vi "Calibrate Probe Tube.vi"(9 "Left":string="ABI-R", 10 "Right":string="SN31", 11 "User ID":string) -> ()   [LabVIEW 2020]
uses:
  epl-vi-lib/Utility VIs/Type Defs/Left-Right ring.ctl
  <vilib>/printing/EasyPrintingControls.llb/layout_options.ctl
  <vilib>/printing/EasyPrintingControls.llb/orientation.ctl
  <vilib>/printing/EasyPrintingControls.llb/panel_scaling_for_page.ctl
  <vilib>/printing/EasyPrintingControls.llb/margins.ctl
  <vilib>/printing/EasyPrintingControls.llb/margin_values.ctl
  <vilib>/printing/EasyPrintingControls.llb/measurement_system.ctl
  <vilib>/printing/EasyPrintingControls.llb/printer_options.ctl
  <vilib>/printing/EasyPrintingControls.llb/printing_method.ctl
  <vilib>/printing/EasyPrintingControls.llb/color_or_monochrome.ctl
  <vilib>/printing/EasyPrintingControls.llb/page_header_options.ctl
  <vilib>/printing/EasyPrintingControls.llb/page_headers.ctl
  <vilib>/printing/EasyPrintingControls.llb/page_header_content_options.ctl
  Type Defs/ACal-Probe Tube Parameters.ctl
  Type Defs/Cal Stimulus.ctl
  <vilib>/printing/EasyPrintingControls.llb/contents.ctl
  epl-vi-lib/Utility VIs/Math VIs/FFT x(t) to dB,Degrees (2D).vi
  epl-vi-lib/Utility VIs/Conversion VIs/Create Waveform Cluster (2D).vi
  SubVIs/Calibration Globals.vi
  <vilib>/printing/EasyPrinting.llb/Easy Print VI Panel or Documentation (refnum).vi
  Instance           1 28Saved   Calibrate Probe Tube .vi
  epl-vi-lib/Utility VIs/Math VIs/dB to Linear (scalar).vi
  <vilib>/Utility/NIReport.llb/NI_ReportGenerationCore.lvlib
panel:
  in  "layout options":T1={"orientation (unchanged)"=0, "panel scaling for page (unchanged)"=0, "margins"={"override VI margins (false)"=FALSE, "margins (1.00)"={"top"=1.0, "left"=1.0, "right"=1.0, "bottom"=1.0}, "measurement system (default)"=0}, "printer options"={"destination printer name (current)"="", "printing method (unchanged)"=0, "color or monochrome (unchanged)"=0}, "page header options"={"page headers (unchanged)"=0, "page header content options"={"Include VI Name"=TRUE, "Include VI Path"=TRUE, "Include Last Modification Date"=TRUE, "Include Date Printed"=TRUE, "Include Page Number"=TRUE, "Include VI Icon"=TRUE}}} {"page header options"."page headers (unchanged)" items=["Unchanged", "Include page headers", "Do not include page headers"]; "printer options"."color or monochrome (unchanged)" items=["Unchanged", "Color/grayscale", "Monochrome"]; "printer options"."printing method (unchanged)" items=["Unchanged", "Standard", "PostScript", "Bitmap"]; "panel scaling for page (unchanged)" items=["Unchanged", "No Scaling", "Scale front panel to fit"]; "orientation (unchanged)" items=["Unchanged", "portrait", "landscape"]; "margins"."measurement system (default)" items=["Default", "US", "Metric"]; "margins"."margins (1.00)"."right" format="%.2f"; "margins"."margins (1.00)"."bottom" format="%.2f"; "margins"."margins (1.00)"."top" format="%.2f"; "margins"."margins (1.00)"."left" format="%.2f"}
  in  "Correction curve":path
  in  "Measure":bool
  out "(mV/Pa)":dbl=40.0 format="%#_4g"
  out "Acoustic System ID":string="SN31"
  in  "Ear":T13
  in  "Probe Mic Gain (dB)":dbl
  in  "Cal Mic Gain (dB)":dbl=40.0
  in  "Stimulus":T14={"Min Freq (Hz)"=50.0, "Max Freq (Hz)"=50000.0, "Freq Step (Hz)"=50.0, "Waveform"=enum."Chirp", "Attenuation (dB)"=30.0, "Sample Rate (Hz)"=100000.0}
  out "Stimulus graph":cluster{i32, dbl, dbl[]}(graph)={0, 0.01, [-5.247460171907412, 0.008605798542191699, -5.263937532639148, 0.024339294749305594, -5.244475767281008, 0.04327175038935926, -5.188768276233243, 0.07159908666817012, -5.095903568565098, 0.11549515149058191, -4.964399941130261, 0.1810884237842581, -4.792264316991073, 0.27442378081433927, -4.577077172797298, 0.40140354945941514, -4.3161060418071555, 0.5677023140763962, -4.0064504089795046, 0.7786503888896317, -3.645220836759635, 1.0390815630417642, -3.2297547859327076, 1.3531417859996795, -2.7578707294700084, 1.724056982991224, -2.22816070014333, 2.153860279401379, -1.6403192706341323, 2.643081666319236, -0.9955040585896162, 3.1904066322148728, -0.2967191285234929, 3.792314555323266, 0.4507918747408072, 4.442712676082995, 1.2391613126860297, 5.132587144315406, 2.057546184165045, 5.849698747965765, 2.8918403003749833, 6.5783571298986745, 3.724486549481605, 7.299313078445633, 4.534431115953833, 7.989813153488007, 5.297265336532347, 8.623863622799167, 5.985602242560379, 9.172750412799761, 6.5697326691648446, 9.605857387646246, 7.018598937096457, 9.891815588212754, 7.301111383534703, 10.0, 7.387813446513752, 9.902367138660988, 7.252873956718745, 9.575595866011744, 6.876350702602797, 9.003455705946067, 6.246627988988914, 8.179282815334176, 5.362884683208197, 7.108396197100778, 4.237401343653944, 5.810239657287673, 2.8974701412652104, 4.3199938484742715, 1.3866355939228834, 2.6893743744841005, -0.235024890715656, 0.9863243167635698, -1.8918657346432832, -0.7066688960181444, -3.49512904116343, -2.2958437123541913, -4.947057814678465, -3.6811314381434963, -6.146708184335848, -4.762782149907513, -6.99733253447503, -5.44942121944958, -7.414996574301741, -5.667084312081226, -7.3378591109482, -5.368539628350952, -6.735306113447965, -4.541978733119788, -5.615921799386064, -3.2179767099964502, -4.033137435294095, -1.4735296001117006, -2.0873657499853566, 0.5679853545614835, 0.0764536954682828, 2.7418756260149975, 2.2766729673521082, 4.8527764144117835, 4.30839594053929, 6.690828848153954, 5.96217634437059, 8.052592456156836, 7.04673009875188, 8.765032133153767, 7.413566916427472, 8.710067062700757, 6.980647540350419, 7.846463408719186, 5.751601312013723, 6.225456709762098, 3.826859567750187, 3.9965653470462574, 1.4034232691160335, 1.4007322096543322, -1.2390126171416238, -1.2507325298668845, -3.7661990085581607, -3.6109846093868825, -5.830158904497616, -5.343446619696167, -7.11863088939354, -6.173269096842483, -7.406665287984586, -5.93697567074002, -6.602097328524571, -4.62149439465155, -4.7759155920390555, -2.383800918156967, -2.1693905978568395, 0.4558663898494483, 0.8275208795869367, 3.4507072628822213, 3.7275911979607788, 6.09235566166205, 6.022996250896586, 7.896571926877759, 7.276660398539333, 8.496267869824582, 7.212524412699896, 7.724300184680044, 5.78609054729564, 5.667189460480745, 3.217206541451461, 2.6736060915361497, -0.028096090734308465, -0.6915362170521967, -3.3109044902910116, -3.7458551362852015, -5.9401233137836575, -5.8269949248777975, -7.320204962233645, -6.442849713395074, -7.095298209127541, -5.400691974640072, -5.2545546954009525, -2.8805696820323017, -2.1668301265948715, 0.5736091158430698, 1.4744009601043935, 4.155120373461428, 4.794822743297185, 6.9746253410301975, 6.946647025249635, 8.282863836240622, 7.332782067475395, 7.681230357484651, 5.788485263093952, 5.259985350440268, 2.6635543896510905, 1.6148842229039682, -1.2321309711394293, -2.2791036731398298, -4.822173581640922, -5.318706845785659, -7.056875219949377, -6.58844576757031, -7.229540772397591, -5.652758866191721, -5.220125424480435, -2.728934669369589, -1.5792762725530691, 1.330004185915103, 2.5947767617377417, 5.26077489392688, 5.97156978417373, 7.7740442713520075, 7.413058271139368, 7.985588198248131, 6.374378980649487, 5.749844302517612, 3.1368042021591003, 1.7656193472640005, -1.2307138864244704, -2.6113675396896427, -5.199351313853099, -5.814263689192346, -7.309114034900627, -6.631386968823555, -6.720768410023753, -4.6897473313856715, -3.5800621548930938, -0.6575552182543789, 0.9704821464587078, 3.946321771794807, 5.176186930576256, 7.302284923331499, 7.337662376963383, 8.011803580119759, 6.514041666961232, 5.706545139116614, 2.967861932299919, 1.272343162390996, -1.8678232780009332, -3.45026885495027, -5.936024879819881, -6.411238921879773, -7.425541450334893, -6.252421914203625, -5.60197735072843, -2.9681759541147814, -1.212009047625889, 2.0072496296359597, 3.7722442843035657, 6.384557487487479, 7.0125100927973065, 8.061414715811145, 6.909383622455292, 6.155974853894271, 3.4311420962567754, 1.5162174765733274, -1.7766786708006803, -3.603327988185656, -6.125870985627785, -6.610596375301682, -7.3634425246130135, -5.9022705997704525, -4.770419048180873, -1.766887564352594, 0.3676255453902768, 3.661744223349101, 5.341314962064073, 7.462373475230487, 7.424660487516245, 7.498419729909054, 5.39409958927202, 3.6620769715753356, 0.30429290403609865, -1.9527130941819373, -4.9937392207499105, -6.143652224116909, -7.419717721833314, -6.423937846193488, -5.477259487880406, -2.545241904374176, -0.2381215906009224, 3.2334674915729873, 5.176970492062233, 7.403858060906316, 7.424812063901678, 7.332703585945119, 5.029648312147353, 2.9739938247968354, -0.5802426219546769, -2.96980091563933, -5.8492898574021845, -6.669677540664699, -7.320605771962078, -5.64372583856975, -3.941020091557808, -0.486803126553241, 2.1098537508064745, 5.382645863920707, 6.752794304321151, 7.939975165779068, 6.746137374430747, 5.3354630175248, 2.0049498872310276, -0.6926053124611669, -4.188393767139286, -5.895140320125075, -7.396021670989176, -6.4835405802843695, -5.2183372128746655, -1.9420199456520648, 0.8323095237238995, 4.436623036483066, 6.288347883410518, 7.866933818470105, 6.992701149290664, 5.66877018952909, 2.3174894102616133, -0.5588466061601974, -4.1880383393350575, -6.003821804112207, -7.419019451098028, -6.328409829492962, -4.734284432309863, -1.1850596867744247, 1.7950178654578355, 5.327091429463836, 6.882140261576732, 7.856640472116676, 6.2803281835987645, 4.22068034616256, 0.3991421081048472, -2.6140204156880023, -5.848350195807402, -6.85636573457159, -7.0910659692341325, -4.7933509719516, -2.1643551542287414, 1.8675265370492249, 4.689874030204529, 7.292308668251718, 7.390111510847516, 6.59199906715598, 3.4336871141493432, 0.30172855553474925, -3.673492374680839, -5.894931811807184, -7.418729223490227, -6.245322255897431, -4.25209871294359, -0.3328874715123917, 2.941917812152746, 6.31946557919589, 7.353133838306091, 7.330124735659604, 4.678678601940708, 1.6295522117378556, -2.5755880072377595, -5.28712450014373, -7.3144555947664305, -6.5735977356081134, -4.770194836178391, -0.8591488588596867, 2.5958602653035596, 6.156976691276675, 7.339590352317998, 7.295293625358333, 4.53266183919819, 1.2891964301376782, -3.0072298175380503, -5.6738166720809495, -7.406990997361928, -6.239496306224862, -3.941192684323301, 0.28294268668459244, 3.772424756570202, 6.9388943995771974, 7.412642145914989, 6.459663864604533, 2.929223388058357, -0.7253749311016806, -4.816256232005783, -6.702620432750113, -7.192902344033079, -4.731369021984241, -1.4414577990167237, 3.0487448569867754, 5.973294402720529, 7.777452265528625, 6.517475422558797, 3.929398783800692, -0.5311427078538121, -4.102206564584618, -6.975532546438933, -6.877235917573633, -5.151749627809858, -1.019946035576886, 2.85574857117119, 6.5142866732599245, 7.426122482652017, 6.575512793162643, 2.9296826424821316, -1.0056189595996894, -5.194472124415492, -6.9244564830663755, -6.869539692795811, -3.7564721469176305, 0.08751061193103099, 4.601488283996679, 6.950180666067047, 7.552463858896631, 4.928522407334323, 1.2339857195152837, -3.467697768024356, -6.260941260422518, -7.362010266767195, -5.130404817874262, -1.5787085489641972, 3.2260063318414076, 6.312999422865575, 7.742481983040587, 5.765824502092311, 2.29686139113806, -2.574183972128345, -5.832423189894068, -7.423361194717821, -5.547501807955327, -2.0757399684555327, 2.8460977007969532, 6.161201434600137, 7.740164989978125, 5.795240360236828, 2.218825065094677, -2.7480716752965813, -6.007130819195174, -7.397987435336653, -5.214791695268458, -1.4420055667696872, 3.5441107546488215, 6.610757652541965, 7.62161758419931, 5.032758273140988, 0.9938080906391938, -3.951552010030123, -6.6595244673234735, -7.090866741949985, -3.9541424698949124, 0.3666032462722816, 5.147025662921905, 7.283044503087227, 6.928843038131749, 3.143361282651853, -1.4005374850137773, -5.81753201637329, -7.131470601307786, -5.810562685267453, -1.3593972322635997, 3.237678001181557, 7.002954174075119, 7.220586802896102, 4.810421693830754, -0.2037693220285648, -4.557771783842997, -7.313595030973062, -6.190231619270408, -2.694006520878864, 2.6098313187672977, 6.2881002013277385, 7.644888179741437, 5.0332073532217505, 0.6422276509988876, -4.487733612052248, -6.96433742668024, -6.595428622107091, -2.5521855587978552, 2.2865678633506223, 6.597316176229779, 7.338285239994512, 5.1022254419284385, -0.016959372200316996, -4.591293583267117, -7.350470455953657, -5.978220674993969, -2.0764227867177043, 3.395236816869554, 6.791143158965057, 7.352228162218951, 3.8427701774074103, -1.0672643055181525, -5.8459021684587515, -7.149031971945431, -5.219227891725583, -0.1004177592343227, 4.6887830076421055, 7.5990316517010985, 6.2070269269780445, 2.115688988887157, -3.4661362625146603, -6.731658881182953, -6.8519111390977505, -2.8522801918666163, 2.2862242384436673, 6.72900730089474, 7.220900563595496, 4.35586130070044, -1.2229073577912795, -5.648862915611157, -7.389024632985817, -4.615740146897012, 0.31918760965121495, 5.5837098321905545, 7.426544277044912, 5.664192513987078, 0.4030823548800622, -4.600945112795148, -7.394431544905614, -5.557595320391062, -0.9370090027809214, 4.704655561012707, 7.339889092334802, 6.2787112720154, 1.2827129427791721, -3.979843266775962, -7.296417113586281, -5.922507567322214, -1.44318806531093, 4.356269929683986, 7.283021687223988, 6.4054972254029865, 1.4203851555677962, -3.947198285633883, -7.304928863219976, -5.849233412081237, -1.2139889713487029, 4.617712545093255, 7.353534406789328, 6.100063253697727, 0.8216317054554423, -4.511552759408483, -7.406095318826852, -5.304382372452656, -0.2405691394206577, 5.428240566118344, 7.425926703045357, 5.243465598093195, -0.5279946590706618, -5.533588570328488, -7.361872248281549, -4.096618104825187, 1.474264963016517, 6.551434833095712, 7.150728253852704, 3.5971745791139096, -2.5716981435457846, -6.655679885547709, -6.719722629272131, -1.9809781668597604, 3.7704867106062423, 7.484853597327619, 5.995321810252248, 0.9693345027842137, -4.9883959449077615, -7.21701623238748, -4.913340447389673, 1.1014843094368336, 6.1077362733100005, 7.418653590903101, 3.4379736602408677, -2.469318380430274, -6.9739072004505465, -6.306633286082643, -1.5808149986014717, 4.647425939667652, 7.407876735275789, 5.4427259675944075, -0.5738915711179777, -5.795510780887788, -7.226577076684699, -3.1818117873187712, 2.853476296586651, 7.275652090831912, 6.283712090560184, 1.2100048808955002, -4.988063124485182, -7.225270522900655, -4.5176796337619365, 1.8444352873823244, 6.631109219631903, 6.992678228704494, 2.0109920015762643, -4.063299376258122, -7.405929161515044, -4.916771011045486, 0.9678524128825984, 6.522515137830295, 6.99560041193589, 2.6271152187851907, -3.948885437252043, -7.192300800581729, -5.2534136062223, 1.0318439544846199, 6.311848705567506, 7.166209195204141, 2.323350785231853, -3.936826451465734, -7.405888659140412, -4.805723062168871, 1.290124743453395, 6.75573752449112, 6.749821833712563, 1.835291400009754, -4.741122013944317, -7.242224259477733, -4.254776132185593, 2.456246771732051, 7.013090118914596, 6.349145545303646, 0.4051417927954177, -5.5188544634287195, -7.226690557563207, -2.765024839084136, 3.729343570414043, 7.554573672535005, 5.035548016008795, -1.2497620581093263, -6.722345116231772, -6.341040872374437, -0.938777516835575, 5.584937372087172, 7.29088401898383, 3.277752823374007, -3.668197539629081, -7.21954700648047, -4.9141953866504275, 1.8607845337324562, 6.881419700776224, 6.414705610677603, 0.3124143648746709, -5.733833290366328, -7.077455525208768, -2.0334400691400996, 4.577687291061455, 7.575544132680769, 3.845466604947863, -2.900155243337663, -7.312647657904366, -5.0325387969350555, 1.4726554460206769, 7.010693797557449, 6.208835270027705, 0.2426368501627138, -6.119786289628639, -6.742878807224529, -1.5366022807910058, 5.358562178640916, 7.291008275054191, 2.986361087280685, -4.181914869472955, -7.27254284643081, -3.9445461493243212, 3.276059924149099, 7.353406806436564, 5.017532453194594, -2.0827734646331777, -6.974967011951131, -5.603801799805588, 1.2479935717871624, 6.790144240279283, 6.3212911871910835, -0.19962218586423452, -6.245716249946395, -6.596693444669236, -0.4520652452418208, 5.971090033733906, 7.044081935464482, 1.2857370221473308, -5.4125325086995915, -7.105320196586026, -1.7178422467752026, 5.1740674229367825, 7.380757371982751, 2.324840249908939, -4.701914033774923, -7.319981402284617, -2.5414947549511457, 4.577072426551161, 7.504757775455616, 2.935040678634225, -4.248566017694976, -7.389068349975114, -2.9525810734921025, 4.277627161008861, 7.534354087203025, 3.1477895890718384, -4.118723423292581, -7.3978556128306145, -2.97682477387077, 4.315562896229031, 7.520352295898593, 2.978030728532146, -4.329172031133085, -7.362041055431735, -2.6157810360379234, 4.686140136961194, 7.443176669474266, 2.413668319234095, -4.853212361187332, -7.226983660393568, -1.8457858961590197, 5.33833667896169, 7.213830229532318, 1.4239626016719844, -5.611417991409709, -6.870925073661793, -0.6360621551866662, 6.158908268204798, 6.680868903172948, -0.012198893040158035, -6.4506233835836015, -6.118102470078314, 1.012431405730744, 6.948896592720228, 5.652805457530667, -1.8568674591179255, -7.121721760234774, -4.774119857796032, 3.007873164854061, 7.407847897177656, 3.950236955566206, -3.9466082818682264, -7.2768739195418695, -2.698095427984128, 5.09842422101464, 7.151880583544878, 1.4998433771111057, -5.9280034587624915, -6.517113218616011, 0.08227476144176188, 6.823062584347205, 5.799336511097809, -1.5342933632456348, -7.237851950393849, -4.522792310107686, 3.233444877508748, 7.537944689067077, 3.148759997984469, -4.624501162666625, -7.193663995647283, -1.274986138271457, 6.025253604588409, 6.58732564498896, -0.5703477954587108, -6.855121697511509, -5.255351399441133, 2.6912635594559378, 7.407826844331432, 3.6548593814698234, -4.483060427885582, -7.134453506819222, -1.447213075625703, 6.166117630160645, 6.383081700870901, -0.7861948037197607, -7.105684033559456, -4.730501596501017, 3.233059875754157, 7.522314740973714, 2.67761848243742, -5.200149255925657, -6.871311330089527, -0.011331621791488056, 6.789393984493315, 5.520727292913766, -2.5675094974361627, -7.3215384228731555, -3.169811702407082, 5.078118913958271, 6.996959773882328, 0.4635379712645482, -6.720929830813573, -5.3743273661307756, 2.5898280055884793, 7.51816284613278, 2.9796279606995535, -5.107951957867861, -6.853606575165182, 0.2145104988875672, 6.948469445520113, 5.082335764255203, -3.2948186891216396, -7.307763003702785, -2.081545339836511, 5.986008904559052, 6.335270153507825, -1.2601441461697336, -7.3037108572907, -3.76436647820519, 4.575386453236491, 7.174988426803019, 0.40886276693731716, -6.718500000770266, -5.156288906754431, 3.3127785405012187, 7.392157940194016, 1.9481390390104314, -6.117936957570988, -5.958154081040177, 2.0133387073918496, 7.4921389318317395, 2.980132608481309, -5.330452107764856, -6.597880522116794, 1.108780699565278, 7.282270450218552, 3.85410194661178, -4.8092811093465295, -6.837333409733931, 0.31368410046975775, 7.203334999165943, 4.277662492602619, -4.3056702174620405, -7.078412185454286, -0.03438186957498213, 7.011907531884418, 4.602962511361689, -4.179018451126646, -7.058557225575194, -0.2457963493496157, 7.06140341649829, 4.540389278552674, -4.138530549108562, -7.106121206873734, -0.015365853308301175, 7.056711255870985, 4.393121269506496, -4.481737357836458, -6.911329938301271, 0.3598426758007237, 7.2690650721030785, 3.8489605944825476, -4.89245298687628, -6.721818960510642, 1.1651210279975381, 7.353013513759481, 3.1608890494445325, -5.6036906401199715, -6.184089002672798, 2.1021341308880115, 7.493896595507685, 2.0161520342524835, -6.251984549771036, -5.482094199600977, 3.3959908559018883, 7.291899898442843, 0.666279618824786, -6.971716416547719, -4.256797330499773, 4.683783173675891, 6.8555516801230185, -1.1236956068984163, -7.3188776276161445, -2.7005285739750873, 6.054328152527586, 5.771774923298172, -2.9959145246337897, -7.320499134142371, -0.5650429875992593, 7.011616036027911, 4.169076331702438, -4.983625449917584, -6.499797553302054, 1.7867319981344782, 7.484495672535726, 1.7913635809048556, -6.515479887937506, -4.9176851263388315, 4.306487294935299, 6.916154946198537, -0.9703314683939835, -7.393387655014362, -2.3237097363788646, 6.309106563315713, 5.298911133350756, -3.943825466303358, -6.961860452300179, 0.8234554913541505, 7.433342869355618, 2.4173152983473027, -6.278708931241014, -5.157599335555851, 4.165978845245447, 6.916269397202499, -1.1368038483555083, -7.417012847519947, -1.8608890143246493, 6.628569163314005, 4.685710151704879, -4.736484110149196, -6.510958460408045, 2.1010756992173847, 7.445750477929317, 0.8291057533600581, -7.02965646602411, -3.587187966152209, 5.735480122805063, 5.772359254023778, -3.4505655445327994, -7.092896487453685, 0.8836811297244362, 7.407655648134268, 1.9307107136610782, -6.719688658193731, -4.279548739125746, 5.170725786787521, 6.204679037376475, -2.996785318715991, -7.172596714740932, 0.49776084697882034, 7.426006530234811, 2.017631158258109, -6.66837225434066, -4.259696555741614, 5.336739235586457, 5.999907565678239, -3.3122677874397706, -7.0790578557442165, 1.130643519486488, 7.426867073907273, 1.2635949671344218, -7.048058314044763, -3.3520919032035184, 6.02307345106183, 5.230819827745236, -4.4800167570289915, -6.480778767262717, 2.5867974703342993, 7.293490166170975, -0.5198521180144519, -7.376174578741273, -1.5422206759324273, 7.016952559870459, 3.4449323971009664, -6.0290299939485195, -5.056927437130529, 4.761619679998125, 6.287895772338952, -3.0893308477577093, -7.079202239575908, 1.374775801813738, 7.414276063661718, 0.4919697724840566, -7.303053345831668, -2.1752733434697866, 6.787874814292458, 3.8020882523454325, -5.925106372577843, -5.087138350895923, 4.789833706094948, 6.18864210441624, -3.4575815730321158, -6.877426298905895, 2.010170539937892, 7.341581121149976, -0.5192665657090618, -7.401020568797851, -0.9455062464022865, 7.262813200154886, 2.330665799263958, -6.782728429921616, -3.5884637749515425, 6.172717552564091, 4.688957650630858, -5.3105372887895905, -5.607877755200963, 4.400303350121803, 6.337379392473475, -3.3307144254223697, -6.872944270575925, 2.2890559166616824, 7.223548472300287, -1.1680785719139684, -7.398264864377694, 0.1334415939306725, 7.416410018479477, 0.9209854360723804, -7.294296784950279, -1.8524520650484861, 7.0556901416999125, 2.765944521584717, -6.7189323138813, -3.5405505538122166, 6.3078322538462475, 4.2783293247911764, -5.839211019870375, -4.8779340722449085, 5.334209601773843, 5.4359950925258325, -4.806197163386051, -5.868145403133641, 4.272409227610091, 6.263089009181842, -3.7421169184660386, -6.551096798996301, 3.228486290643495, 6.810854343669898, -2.7369035091718157, -6.985435068214615, 2.276956012631502, 7.141965492640768, -1.8508271751906238, -7.235045328152592, 1.46532362307337, 7.319233862104875, -1.120278634308993, -7.359869430159808, 0.8205755195832674, 7.398364006797049, -0.5645229317121275, -7.410371912701982, 0.3558454834427866, 7.423874712291961, -0.19201220967215066, -7.424655369356793, 0.07618030599874454, 7.427157166498761, -0.005469421733202465, -7.427230463015562, -0.01714716141569475, 7.42575399924954, -0.0053761002394784535, -7.428634215170117, 0.07599364351345202, 7.423183005309935, -0.19173233891843405, -7.425362887881296, 0.35547256648551373, 7.4089212073272375, -0.5640576747585542, -7.3998878507086365, 0.8200189260273955, 7.35847182632419, -1.1196328593441274, -7.320831555676253, 1.4645915959194222, 7.233745459785213, -1.8500137808532942, -7.143687660520191, 2.2760675624765674, 6.984288856136283, -2.735949217361889, -6.812761209684803, 3.227477546164284, 6.550167413273623, -3.7410689909103785, -6.265244901517009, 4.27134025432215, 5.867496052705217, -4.805129973770331, -5.438459285250389, 5.333170283282182, 4.877616717905038, -5.83823069799834, -4.281142526192145, 6.306945050488885, 3.540590198072637, -6.718176876739951, -2.7691111567212734, 7.05510677865644, 1.8528274290289084, -7.293928528267814, -0.9244533752976082, 7.4162987415759165, -0.132818336985834, -7.398451730141151, 1.1644369953415918, 7.224068954342528, -2.288355223399794, -6.873828011689916, 3.3271136589993873, 6.338644297302056, -4.399782504607134, -5.609529600364011, 5.307273332538398, 4.690983798162676, -6.172703613171116, -3.590833312033117, 6.780147752037883, 2.333323888376624, -7.263656143383226, -0.948376032135294, 7.399456530337989, -0.5162875524339932, -7.343573759427886, 2.0072051922935303, 6.877104314241444, -3.4547732535611546, -6.19191412499727, 4.787336461080588, 5.088064593730297, -5.923080493918324, -3.806497651280201, 6.786472135171221, 2.1771391413601497, -7.302408840932891, -0.4970322216789631, 7.4144898134942485, -1.3726265822772437, -7.080329883784682, 3.0844236539756817, 6.289931255332871, -4.760110006045242, -5.059797647129997, 6.025259581286349, 3.448486988188797, -7.017048997819728, -1.5462376697209068, 7.374405141929314, -0.515662877445445, -7.295859359789407, 2.5827723313479654, 6.481385192945382, -4.476517940242472, -5.235462646037644, 6.0204507306915565, 3.354643120470073, -7.046616127697511, -1.2696273237792064, 7.42681906050643, -1.127457940232792, -7.080495585247652, 3.306500997165923, 6.002766494492259, -5.334780914164535, -4.263747781980172, 6.664750626009611, 2.022480594483122, -7.426949012757776, 0.49263877679293694, 7.17235199964729, -2.9920030389433516, -6.209096050999331, 5.166905137167382, 4.282435540599078, -6.717382532006223, -1.9374669609565376, 7.407253702447325, -0.8796397991271134, -7.094554372923783, 3.444106102793002, 5.775939653753163, -5.733266194931018, -3.592253837019415, 7.026405408350863, 0.8349480400453515, -7.447737561133129, 2.09534544545967, 6.512304597813737, -4.731810644145896, -4.691959785589022, 6.62578766384903, 1.8654096452406224, -7.416694437351456, 1.129108339115356, 6.918579662084281, -4.162131840100958, -5.162231198965337, 6.2738377553254665, 2.4234912578716203, -7.434087491324242, 0.8168691413127844, 6.9625731321676385, -3.9381305832087077, -5.305175618692445, 6.305508388999558, 2.3287308778455165, -7.39273333221167, 0.9619683348921999, 6.918703016090921, -4.302183403773263, -4.922998417302366, 6.510675562341595, 1.7983364322760444, -7.485960450584175, 1.7796646687065727, 6.501756309519529, -4.978157283984076, -4.176730609481952, 7.009149341278814, 0.571052691676939, -7.321768717118409, 2.987504426221774, 5.776587877050262, -6.051253172668277, -2.7077435875394817, 7.316534680634138, -1.1159462505698252, -6.860213533626597, 4.677623140441568, 4.261808797028619, -6.968947336445471, -0.6758019546077514, 7.293437803342252, -3.390165972287008, -5.4876318472838115, 6.2461631977725816, 2.0241446125112845, -7.4954119353173665, 2.0940759522437595, 6.187167758336899, -5.598114292790371, -3.1701275033281733, 7.351797337504524, -1.1580580802763034, -6.725505313751188, 4.884481308744809, 3.8564603654920004, -7.268363258796754, 0.3509859330417606, 6.912882810353109, -4.474590682398902, -4.401919906179307, 7.053881749985286, 0.022988448800186856, -7.108773997326044, 4.129480344469301, 4.547697255690019, -7.059723053721764, -0.2551245805506439, 7.059680792385098, -4.171223699204117, -4.611945558386291, 7.008762407642546, 0.042470663314095713, -7.081315557630775, 4.2963933331143425, 4.285592968508252, -7.202048473201601, 0.3038923316421848, 6.839434863403917, -4.801739350059988, -3.864136012017699, 7.280300005462442, -1.100319512200232, -6.602501910121454, 5.322037732448754, 2.989447224049214, -7.492893646869789, 2.0034541893218076, 5.962668338777362, -6.112059145100089, -1.9596868346605159, 7.3931639559278555, -3.3047948125244133, -5.163874183028224, 6.712774702292517, 0.41948497251843697, -7.179651304541224, 4.566926328514163, 3.7721017633222043, -7.301742938608468, 1.247974714653711, 6.340961932698631, -5.9808100328068114, -2.0921150883882254, 7.307239632493462, -3.2848626127685425, -5.092066037197858, 6.944504984781181, -0.20474190955431903, -6.857948843428377, 5.098375833844543, 2.990053475182424, -7.519297579123885, 2.5790650682322824, 5.380641776032993, -6.715999006321392, -0.4766188663610665, 7.000863251799099, -5.070901008731789, -3.180442871449945, 7.3195245653301555, -2.5563852601331076, -5.530328479134261, 6.784541075758663, 0.021846766029578427, -6.875870748801165, 5.19020057592572, 2.6889310631973586, -7.524267826482181, 3.222047600888891, 4.738337868478731, -7.102092994604997, 0.7724403891886568, 6.389418263773441, -6.160387201523187, -1.459478075988101, 7.135769908395196, -4.4730101181799045, -3.6674390146075444, 7.4068998598456695, -2.680792754051274, -5.264378563255567, 6.8491697160324865, -0.5575064840759716, -6.595111165912422, 6.017658233787291, 1.2862991316369836, -7.196900286925187, 4.612915273325978, 3.1606725654779995, -7.539482019353017, 3.2215078866958375, 4.531700522411171, -7.234851524908173, 1.5197555563401193, 5.807722455458481, -6.818743669479842, 0.06874191811179253, 6.521738478319468, -5.919786523848885, -1.5147501872859683, 7.155568020219869, -5.089681973749451, -2.7109603599788237, 7.27667821145293, -3.934822470750932, -3.9636585033284337, 7.406825360953803, -2.9964038113230105, -4.78490694433085, 7.1170984144646665, -1.8431296498239582, -5.663768656202124, 6.943841635253259, -0.9996830447815409, -6.126239135094078, 6.44242538231895, 0.0022661839074547474, -6.689148614238921, 6.150758430711532, 0.6491137587774676, -6.876473690356764, 5.600597037938297, 1.438431378236845, -7.219716927533895, 5.32800788552948, 1.858656623567726, -7.230408849302793, 4.84061743918104, 2.4278729447225573, -7.447263467847703, 4.674399499851773, 2.6283900709131776, -7.3640282309582075, 4.315486817425743, 2.992045282935633, -7.523390082580188, 4.303019677466001, 2.989368019667606, -7.399202672469594, 4.104499863871741, 3.1618987508963645, -7.537176064176618, 4.264799022449545, 2.965399091516734, -7.39063683180584, 4.234314619589935, 2.949607691346328, -7.508249288816504, 4.564492323474465, 2.5549391062473332, -7.322675857688303, 4.688220682057052, 2.340168464155817, -7.385834829248802, 5.162403783463528, 1.732128463925866, -7.110055992690154, 5.400174794944171, 1.3019109227170205, -7.05163839036323, 5.9612505643602445, 0.46710003258039723, -6.6043089484332125, 6.235743883185024, -0.1829227657568783, -6.3320645085950025, 6.78331932492377, -1.2328061845999947, -5.614873557507866, 6.968691662259254, -2.0664648083747257, -5.031861790195274, 7.350986726369583, -3.2619903508673036, -3.9590863704478507, 7.27136238791224, -4.167636243486004, -3.0038333371520984, 7.294295183317757, -5.347603856785915, -1.553673636572424, 6.747862476502382, -6.109829647955342, -0.2617036301608677, 6.2184968509740735, -7.005329076788003, 1.4552699482895806, 5.043760944872093, -7.3095157960751225, 2.882386539798747, 3.86078493627221, -7.578060173790286, 4.5634885893059804, 2.0492093738664683, -7.08292207485835, 5.721307226434584, 0.3305956155972155, -6.426019657561329, 6.87451611844762, -1.84439975171717, -4.92796616455454, 7.216134662172068, -3.6521194269538917, -3.296042654826917, 7.294400492737467, -5.573654506029841, -0.9572913111545998, 6.348543917775765, -6.714350580421591, 1.2298238259910688, 5.04938878832608, -7.553945454293956, 3.7129464338939493, 2.7809817034388855, -7.231056372723618, 5.505106297311093, 0.42424361211661904, -6.361264831276551, 7.006737013250193, -2.439371902402299, -4.270596708720245, 7.241505567361612, -4.726164670376518, -1.8557306482234468, 6.757935482804603, -6.7480969586471, 1.2708184123790633, 4.81878599994673, -7.404389234655259, 3.918913357156455, 2.3421345932955466, -7.174422736038775, 6.3013486152791, -1.0135204245187428, -5.267512589575221, 7.188534157845813, -3.9318776684931467, -2.6475785675015215, 7.002344494894086, -6.513412931662251, 0.9477685116477176, 4.930013829280428, -7.404379701622458, 4.045094340786787, 2.0306593181891355, -7.002367279442268, 6.621835978662278, -1.8258397362624548, -4.534033458089634, 7.224602677252942, -4.97269404183121, -1.2320477316455334, 6.294781517920667, -7.270778122603829, 2.8341632946516633, 3.198978124750698, -7.231391423808875, 5.781593017575835, -0.5528605758650056, -5.459158003220313, 7.4063281953931135, -4.631871853515469, -1.601600262943367, 6.315389847394693, -6.966529773901621, 2.447850744710138, 3.4569861922628107, -7.425240673390551, 6.095444184751662, -1.0815069300039253, -4.929556591440002, 7.215639408353774, -4.972264895553426, -0.9924847782794413, 6.008185400083194, -7.4818575849958755, 3.7515742001815027, 2.000490718543498, -6.729073025424236, 6.64579440736328, -2.550936603096015, -3.6183706182232376, 7.156697145515479, -6.541256852987952, 1.4523963409777605, 4.1133142458405665, -7.364794926851754, 5.51789649365079, -0.505557176160088, -5.261523967685936, 7.426258928041062, -5.413546798120738, -0.263235157814853, 5.318053870586352, -7.4043596589994065, 4.492482678274301, 0.844352857034492, -6.115537395358456, 7.350280323270243, -4.6006069887787335, -1.2367253215057632, 5.8609954617576125, -7.3007165912202545, 3.92653119050302, 1.4431880652798892, -6.419893604268694, 7.2784158512998705, -4.338275415375522, -1.4661598110978695, 5.934118913683494, -7.291991563704478, 3.958950664748876, 1.305963864342815, -6.293925752666992, 7.336234811203122, -4.687123985852185, -0.9606126730331556, 5.570984052327365, -7.392161468057767, 4.581301695092964, 0.4270305896089277, -5.682073935741933, 7.4262938029902, -5.5683777501965395, 0.2950364452285744, 4.632540459249535, -7.391433011418179, 5.632586262553019, -1.1988740828766566, -4.377654612826481, 7.226579729538144, -6.718450445829406, 2.262858753334338, 2.8731247253419645, -6.861379048083197, 6.721788759174529, -3.4442429483303, -2.14114457261647, 6.220624200353356, -7.596652158882762, 4.669432578779883, 0.12387692375389034, -5.236992463434808, 7.149084332880998, -5.830382883881306, 1.0410380798767536, 3.8643120403514413, -7.361226465593431, 6.7808670309515096, -3.3737095944247493, -2.1007829704785723, 5.99045721807297, -7.34677816766543, 4.570498185601873, 0.008613672596484849, -5.1231358843378425, 7.342191617399275, -6.585259614011678, 2.2620478527090846, 2.574553805673502, -6.607273960670142, 6.9570939290320055, -4.467031622868547, -0.6696608618019022, 5.052324327106797, -7.649743843598196, 6.274158172352818, -2.5864289592375957, -2.7184277658270983, 6.201577041856491, -7.3089648517917825, 4.536286597181077, -0.17736446399596073, -4.8328595514011345, 7.226742983588233, -6.993014288537623, 3.2137210986872775, 1.3838896103754983, -5.827148554402899, 7.129947624107842, -5.800840769478473, 1.3729310187592958, 3.1676946513050668, -6.942410035578347, 7.277720324031, -5.127992439988434, 0.33957055186316665, 3.974855609274266, -7.098896736644328, 6.648556419109189, -3.928448266747144, -1.0224589472135093, 5.052834982863984, -7.627831099689657, 6.598212026349369, -3.5208177769270548, -1.469001455707609, 5.2316972628351, -7.400380144351477, 5.991093989831807, -2.7222982355420977, -2.247125274400901, 5.812594418939864, -7.7427233018528705, 6.145580670964048, -2.821265821434809, -2.102605496007431, 5.563161626582352, -7.424209577944001, 5.815177136752605, -2.5477237929533865, -2.3255424622827627, 5.783608358808926, -7.745679498267217, 6.298014094539757, -3.2012855156352287, -1.6065085533261036, 5.148197704668377, -7.3657296410551485, 6.246286236890397, -3.442330560665203, -1.2639417779734765, 4.949991585873638, -7.560775044882288, 6.939971191850884, -4.579261804509102, 0.05858411924960321, 3.779123600247425, -6.880518934336202, 6.917040353601821, -5.173614763480565, 0.9754609373700446, 2.956506600714473, -6.592912141972517, 7.4258189084584085, -6.499306327430656, 2.8285933864815798, 1.047396122123962, -5.1729490368667586, 6.882326856563093, -6.965310319077968, 4.077020492657918, -0.5015307010060882, -3.956922458816071, 6.531699352884887, -7.776811366439418, 5.955507236501781, -3.0222961221574667, -1.4708296934614629, 4.751648719123602, -7.200330384846797, 6.691981343928857, -4.7932614113136305, 0.6940370291419778, 2.956991366449558, -6.478487982384133, 7.41442217295258, -6.926029486606039, 3.746193231842714, -0.2539470394846976, -3.967021195040008, 6.251749853525533, -7.4046460924651285, 5.654604556031489, -2.979120396374964, -1.3211889697237222, 4.557025442790835, -7.308144738886594, 7.3348313379395815, -6.138848324146861, 2.5668157793901107, 0.8882457301232092, -4.79396810354764, 6.582694652151162, -7.308962004789193, 5.265573222339429, -2.54623072019011, -1.6619016600411323, 4.702996543496684, -7.34299820504679, 7.348679944072046, -6.301756301900259, 2.912937368325551, 0.362837300700869, -4.277992932439985, 6.257722311250287, -7.417090175268114, 5.876733812361009, -3.645787054978731, -0.33506782078237074, 3.461965963942266, -6.611286905350711, 7.393194842073476, -7.281372738476794, 4.664950328748116, -1.8374308885384962, -2.1951255396175178, 4.8146900090927485, -7.1006011117078724, 6.848978759475313, -5.828316029691708, 2.5829805203545937, 0.43158173613830925, -4.250149129708139, 6.297659381527943, -7.860910136874013, 6.869818954407151, -5.303798097092393, 1.7632278811122357, 1.2155574943688954, -4.759540178375289, 6.340122881958311, -7.417312754207814, 5.986144172937015, -4.16069442657965, 0.5246046416014631, 2.3489569747076167, -5.693929552737952, 7.003825084669513, -7.864691027681262, 6.270581742742224, -4.409792936038569, 0.7991170110753397, 1.97213524398193, -5.242113557016021, 6.49346196345197, -7.392805536911185, 5.876502286494598, -4.160505865130327, 0.6578267192883152, 2.0374763679515113, -5.362595272327349, 6.760241212561402, -7.941376744791632, 6.738615836392951, -5.358361147182795, 2.077192239968285, 0.5191192688925419, -3.9699143045716863, 5.661231585117198, -7.326320600203067, 6.659725626219334, -5.828032675361544, 2.9379742147542807, -0.5458802351538145, -3.0080158388942864, 5.055017893867966, -7.3481262513305845, 7.425119819950367, -7.391905633350139, 5.152052923029143, -3.20248238397998, -0.27288734698164785, 2.5754074887880556, -5.500754902496265, 6.434232200829689, -7.417890885677318, 6.127114162366173, -4.967673000031969, 1.9181756054066286, 0.33947319724950403, -3.695562055299864, 5.418308414317603, -7.512708357590764, 7.4243142218918905, -7.450335338192585, 5.31665400343499, -3.6308323615766187, 0.3321398230231999, 1.79914116656524, -4.7976635210734795, 5.917922990275773, -7.368061649105391, 6.600712569894668, -6.105486129243958, 3.5722882353210865, -1.74173015644146, -1.5533898200158465, 3.463083883106812, -6.181473966913003, 6.92255847897142, -8.063486649740032, 7.000574489191534, -6.362960118523379, 3.740975055094738, -1.9729599665011293, -1.2478633659399847, 2.998482256910706, -5.625837740919566, 6.264219153614564, -7.426596722780991, 6.398613544129925, -5.913844377509871, 3.4182159381994284, -1.8321580021758126, -1.3105004576865906, 3.0016636662514258, -5.735158441688524, 6.531739569970374, -8.019546640911276, 7.331994466370419, -7.286645112735421, 5.149556171457292, -3.9142671796692436, 0.9336116352886903, 0.6927158330188999, -3.612672995234601, 4.7137959754242935, -6.73658179371383, 6.6346571947790824, -7.302209593913814, 5.795068501449539, -5.172343584324118, 2.5762835163537656, -1.1934421917001579, -1.804468492654923, 3.171088355631257, -5.7793003656119355, 6.393784309414009, -7.996049229345152, 7.411060370892994, -7.762557498808378, 5.948958347728496, -5.231718365678255, 2.5590674075491497, -1.2933333636387538, -1.6165629767290817, 2.7611072801118337, -5.247271942913456, 5.670032540312404, -7.238248279520735, 6.585217567275997, -7.0446006808992525, 5.29561152171372, -4.792602259262475, 2.2425269594214385, -1.1938112847959148, -1.6549067841050247, 2.6998589046144614, -5.2927446310950454, 5.812870310423772, -7.698292293713049, 7.3388236732487755, -8.28019598300212, 6.932910914940819, -6.9534162389356515, 4.764972257948207, -4.121203823492364, 1.4360094015377518, -0.5357722872155042, -2.204341640419693, 2.9128690389473446, -5.282266228656416, 5.419591731393694, -7.106839860224447, 6.4438021304455715, -7.313059986369838, 5.809598972571791, -5.915965939957716, 3.713706626485786, -3.2749969843658926, 0.6512300911768543, 0.012026951770659284, -2.714019987392237, 3.253414807170112, -5.69991845017277, 5.8113132432249195, -7.743324131730205, 7.2220557533050425, -8.498380450091945, 7.268899630789249, -7.881800176248844, 5.99954486150076, -6.063748999136739, 3.692761927651043, -3.4136061127888384, 0.787414151244069, -0.41684012306177026, -2.2080310034069353, 2.41812472939367, -4.806846768252448, 4.645499889116734, -6.620531848055124, 5.946865109984115, -7.409905347313126, 6.167509800001608, -7.106322017952566, 5.322833865617136, -5.804172009452375, 3.578359262439368, -3.7302051938133314, 1.2104385444748584, -1.1978513115225842, -1.4435399239016196, 1.444467731214275, -4.03664782410229, 3.8627627119142764, -6.25815082231989, 5.778194335534294, -7.86819819366995, 6.995042836043658, -8.718691134212639, 7.414384035235543, -8.759938452079965, 7.034122922408689, -8.034654277369544, 5.937686580174754, -6.66218128204142, 4.27467462474421, -4.8164904448940336, 2.2371199399618695, -2.701575755643038, 0.03482568895657347, -0.5274594690958865, -2.1273331461358005, 1.5106872433618135, -4.068058156254445, 3.248659237728493, -5.643013827979403, 4.563778945895203, -6.752559806240499, 5.379874073549703, -7.344117745090801, 5.667232207973067, -7.4099562403169825, 5.438488776356751, -6.981474683255755, 4.741607705078281, -6.121181718514305, 3.651149172940014, -4.913528823321419, 2.258923894463806, -3.4556155395432104, 0.6649510738346807, -1.848572613500148, -1.0305914032602168, -0.1901912425558332, -2.733975688884164, 1.4308680272693648, -4.362866739420549, 2.939162059221394, -5.849564580716037, 4.2748922584254565, -7.142658578097501, 5.394840885380697, -8.207307420849304, 6.272064382064025, -9.024416547026506, 6.894630119268244, -9.5890056878368, 7.263688328002469, -9.908051054644872, 7.391151456906446, -9.998057878090384, 7.2972171142584985, -9.882577511138726, 7.007925584853289, -9.589835991403676, 6.552894832008215, -9.150593256340626, 5.963329577900592, -8.596308038360473, 5.270359691520895, -7.957645334925064, 4.503728562004171, -7.263332529784905, 3.690825157328008, -6.539347046865433, 2.8560339911230104, -5.808402456077195, 2.0203645938053025, -5.089690371579313, 1.2013153113285906, -4.398831191514963, 0.41292417935108783, -3.747986546005382, -0.3340389300936554, -3.1460891079710174, -1.0317808083548137, -2.5991501575889053, -1.675130603661785, -2.110611116054271, -2.26115317117216, -1.681711496311775, -2.7887543416584526, -1.3118518513170483, -3.258296483154118, -0.9989359869066474, -3.6712374371795624, -0.7396817348255229, -4.029801374122101, -0.5298938491852471, -4.336686396649448, -0.36469607667446163, -4.594810821693589, -0.2387221959712173, -4.807097939171929, -0.14626790161355924, -4.976297598812266, -0.08140691971884682, -5.104842120199285, -0.0380757927960068, -5.194733656386892, -0.010132461927248428]}
  in  "Averages":i32=256
  in  "Cal Mic Sens":dbl=-146.12351367888365 caption="(dB V/SPL)" format="%.2f"
  in  "RETURN":bool
  in  "START":bool
  in  "STOP":bool
  out "finished":errorcluster
  in  "Data tabs":enum32{"Raw", "Calibration"}(tab)
  out "Mic signals":cluster{"offset":dbl, "dx":dbl, "Y":dbl[][]}(graph)
  out "Mic mag":cluster{"offset":dbl, "dx":dbl, "Y":dbl[][]}(graph)
  out "Acquired":i32=1
  out "PT mag":cluster{"PTC Mag":dbl[], "PTC Phase":dbl[]}[](graph)
  in  "Open Button":bool
  in  "Clear Button":bool
  in  "Smooth Button":bool
  in  "Validate Button":bool
  out "Path":path
  out "PT phase":cluster{"PTC Mag":dbl[], "PTC Phase":dbl[]}[](graph)
  out "Mic phase":cluster{"offset":dbl, "dx":dbl, "Y":dbl[][]}(graph)
  # "Calibrated Mic Sensitivity"
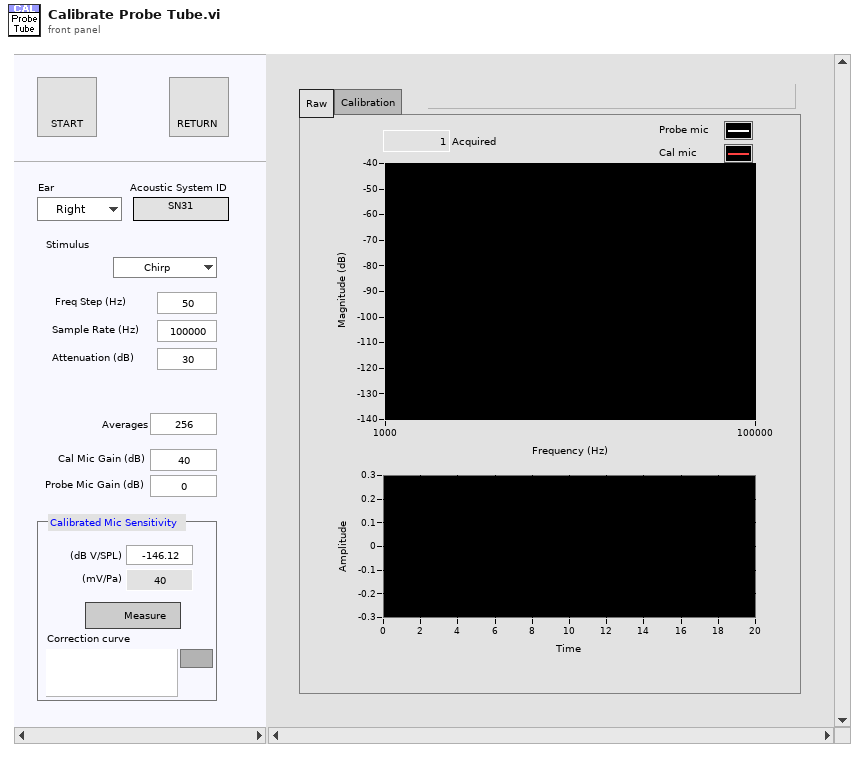
[diagram p1: front panel]
types:
  T1 = typedef "NI_ReportGenerationCore.lvlib/layout_options.ctl" = cluster{"orientation (unchanged)":T2, "panel scaling for page (unchanged)":T3, "margins":T4, "printer options":T7, "page header options":T10}
  T2 = typedef "NI_ReportGenerationCore.lvlib/orientation.ctl" = u16
  T3 = typedef "NI_ReportGenerationCore.lvlib/panel_scaling_for_page.ctl" = u16
  T4 = typedef "NI_ReportGenerationCore.lvlib/margins.ctl" = cluster{"override VI margins (false)":bool, "margins (1.00)":T5, "measurement system (default)":T6}
  T5 = typedef "NI_ReportGenerationCore.lvlib/margin_values.ctl" = cluster{"top":dbl, "left":dbl, "right":dbl, "bottom":dbl}
  T6 = typedef "NI_ReportGenerationCore.lvlib/measurement_system.ctl" = u16
  T7 = typedef "NI_ReportGenerationCore.lvlib/printer_options.ctl" = cluster{"destination printer name (current)":string, "printing method (unchanged)":T8, "color or monochrome (unchanged)":T9}
  T8 = typedef "NI_ReportGenerationCore.lvlib/printing_method.ctl" = u16
  T9 = typedef "NI_ReportGenerationCore.lvlib/color_or_monochrome.ctl" = u16
  T10 = typedef "NI_ReportGenerationCore.lvlib/page_header_options.ctl" = cluster{"page headers (unchanged)":T11, "page header content options":T12}
  T11 = typedef "NI_ReportGenerationCore.lvlib/page_headers.ctl" = u16
  T12 = typedef "NI_ReportGenerationCore.lvlib/page_header_content_options.ctl" = cluster{"Include VI Name":bool, "Include VI Path":bool, "Include Last Modification Date":bool, "Include Date Printed":bool, "Include Page Number":bool, "Include VI Icon":bool}
  T13 = typedef "Left-Right ring.ctl" = enum16{"Right", "Left"}
  T14 = cluster{"Min Freq (Hz)":dbl, "Max Freq (Hz)":dbl, "Freq Step (Hz)":dbl, "Waveform":enum16{"Chirp"}, "Attenuation (dB)":dbl, "Sample Rate (Hz)":dbl}
  T15 = typedef "ACal-Probe Tube Parameters.ctl" = cluster{"Ear":T13, "Stimulus":T16, "Averages":i32, "Cal Mic Gain":dbl, "Probe Mic Gain":dbl, "Cal Mic Sens":dbl, "Correction":path}
  T16 = typedef "Cal Stimulus.ctl" = cluster{"Min Freq (Hz)":dbl, "Max Freq (Hz)":dbl, "Freq Step (Hz)":dbl, "Waveform":enum16{"Chirp", "Weighted"}, "Attenuation (dB)":dbl, "Sample Rate (Hz)":dbl}
  T17 = typedef "NI_ReportGenerationCore.lvlib/contents.ctl" = u16
  T18 = cluster{"Probe Tube Cal Path":path, "Params":T15}
  T19 = typedef "TDT-Device Config.ctl" = cluster{"Output":T20, "Input":T22}
  T20 = typedef "TDT-Output source.ctl" = cluster{"Device":T21, "Num":i32}
  T21 = typedef "TDT-Device ID.ctl" = enum16{"None", "PA5", "RP2", "RL2", "RA16", "RV8", "RX5", "RX6", "RX7", "RX8", "RZ2", "RZ5", "RZ6"}
  T22 = typedef "TDT-Input source.ctl" = enum16{"Front Panel", "RA4LI", "RA16LI"}
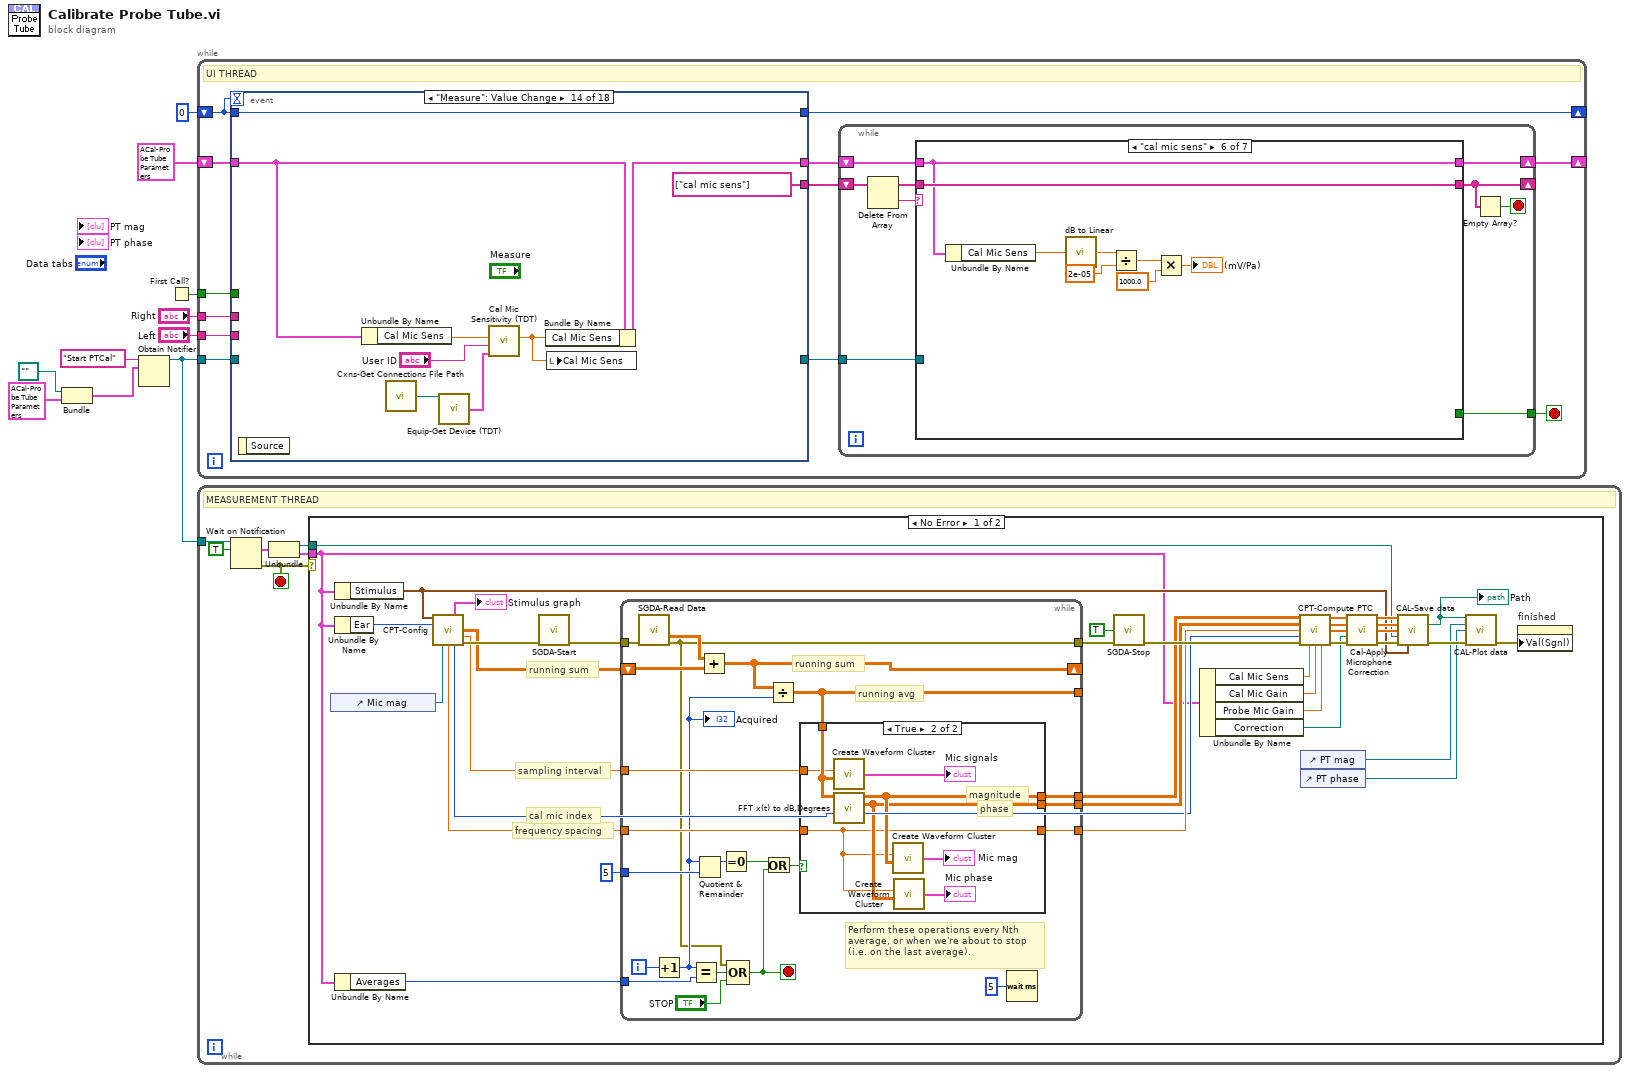
[diagram p0: block diagram]
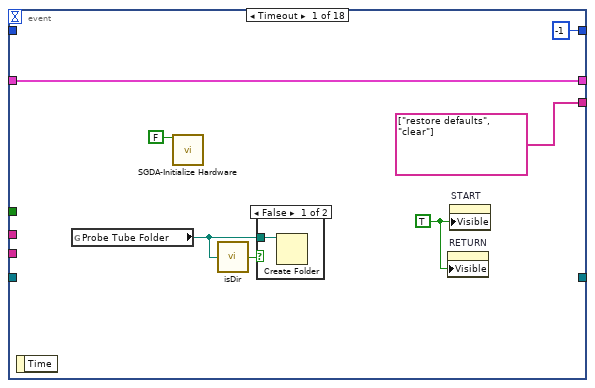
[diagram p2: hidden frame]
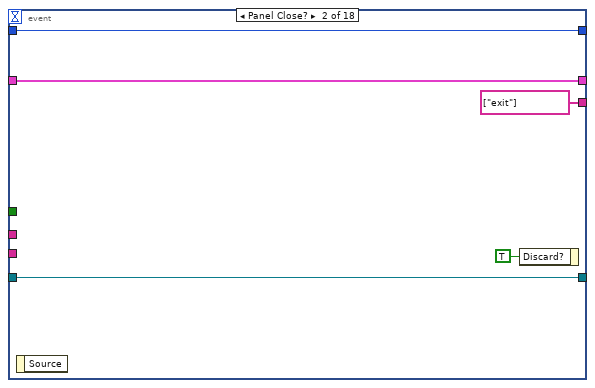
[diagram p4: hidden frame]
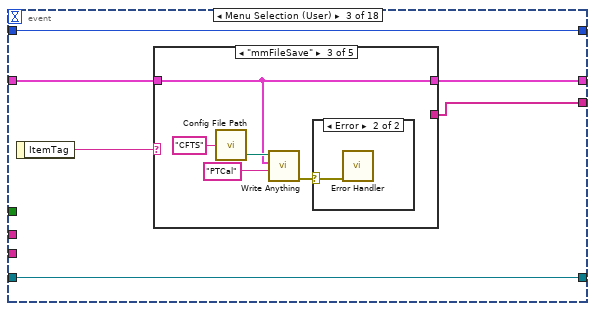
[diagram p5: hidden frame]
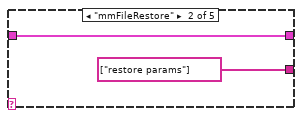
[diagram p7: hidden frame]
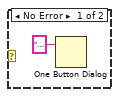
[diagram p8: hidden frame]
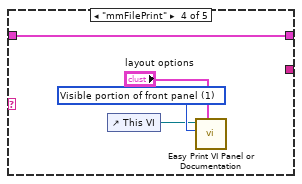
[diagram p9: hidden frame]
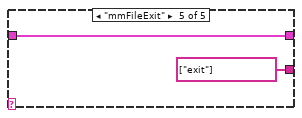
[diagram p10: hidden frame]
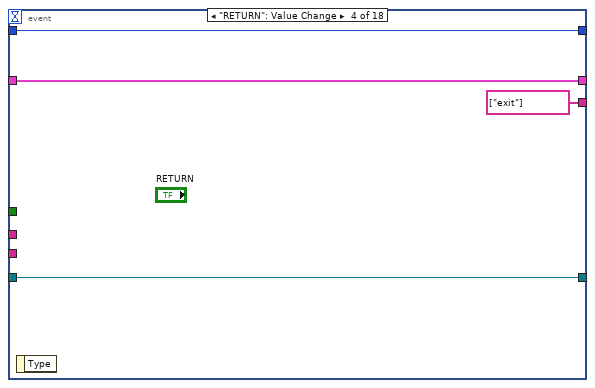
[diagram p11: hidden frame]
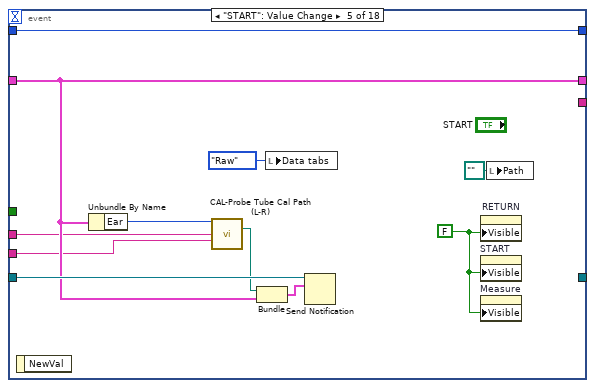
[diagram p12: hidden frame]
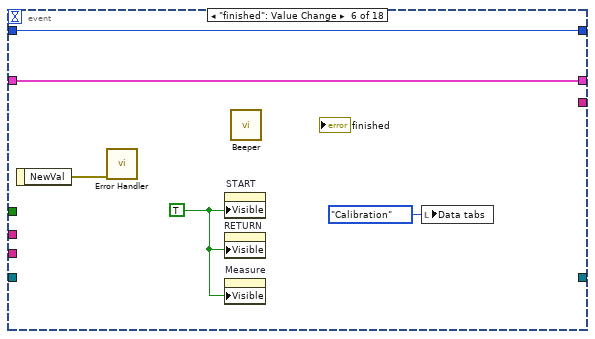
[diagram p13: hidden frame]
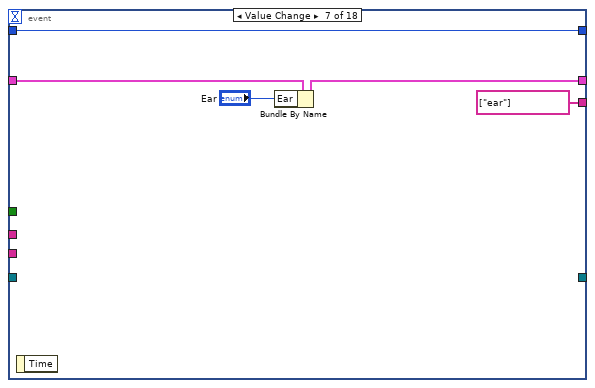
[diagram p14: hidden frame]
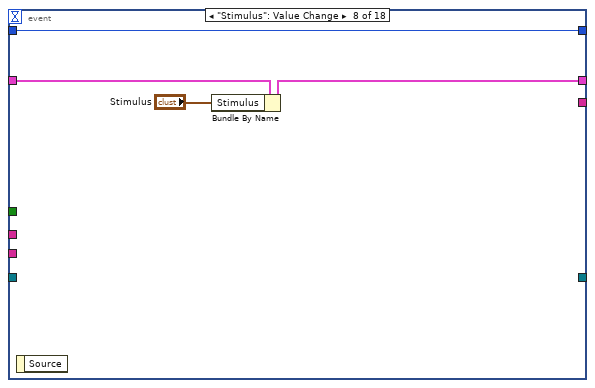
[diagram p15: hidden frame]
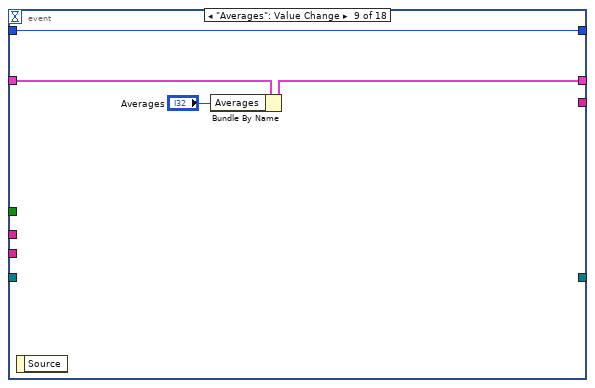
[diagram p16: hidden frame]
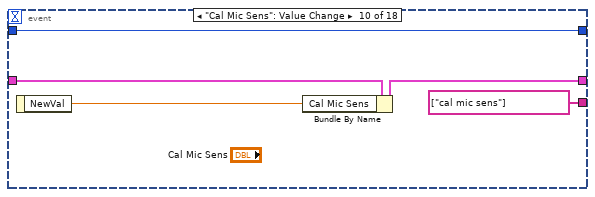
[diagram p17: hidden frame]
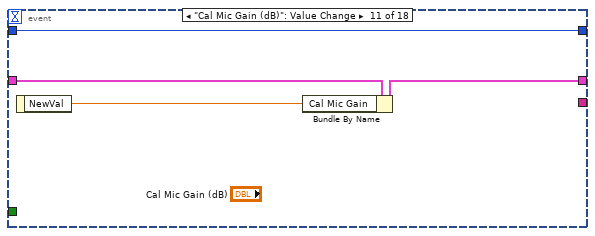
[diagram p18: hidden frame]
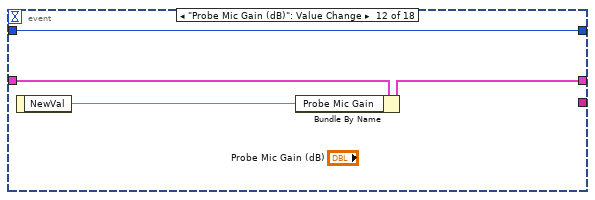
[diagram p19: hidden frame]
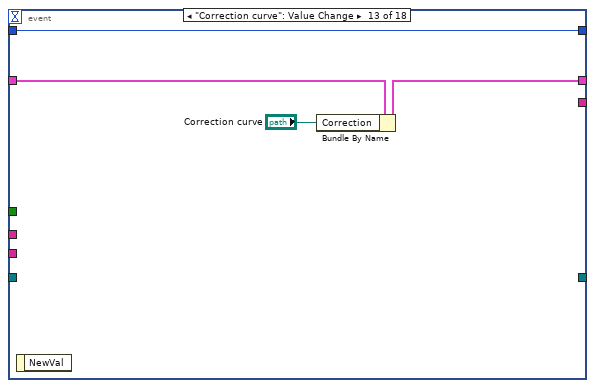
[diagram p20: hidden frame]
diagram:
  n1 = Bundle(path "", "Params"=T15 {"Ear"=enum."Right", "Stimulus"={"Min Freq (Hz)"=50.0, "Max Freq (Hz)"=50000.0, "Freq Step (Hz)"=50.0, "Waveform"=enum."Chirp", "Attenuation (dB)"=20.0, "Sample Rate (Hz)"=100000.0}, "Averages"=0, "Cal Mic Gain"=0.0, "Probe Mic Gain"=0.0, "Cal Mic Sens"=0.0, "Correction"=path ""}) -> (w1:cluster{path, "Params":T15})  [unwired: 1 in]
  n2 = Obtain Notifier(name (unnamed)="Start PTCal", notification data type=w1) -> (notifier out=w10:refnum<notifier>)  [unwired: 2 in, 2 out]
  n3 = First Call?() -> (First Call?: T/F=w7:bool)
  n4 = while {
    tunnel: w10 -> [w22]
    shift-right: [w21] -> _
    shift-left: 0 -> [w17]
    tunnel: w7 -> [w20]
    tunnel: "Right" -> [w19]
    tunnel: "Left" -> [w18]
    shift-right: [w11] -> _
    shift-left: T15 {"Ear"=enum."Right", "Stimulus"={"Min Freq (Hz)"=50.0, "Max Freq (Hz)"=50000.0, "Freq Step (Hz)"=50.0, "Waveform"=enum."Chirp", "Attenuation (dB)"=20.0, "Sample Rate (Hz)"=100000.0}, "Averages"=512, "Cal Mic Gain"=40.0, "Probe Mic Gain"=40.0, "Cal Mic Sens"=-156.0, "Correction"=path ""} ("Params") -> [w12]
    stop <- w14 stop-if-true
    # "UI THREAD"
    n5 = event shown="[13] \"Measure\": Value Change" {
      selector: _ -> [_ _ _ _ _ _ _ _ _ _ _ _ _ _ _ _ _ _]
      dyn-events: _ -> [_ _ _ _ _ _ _ _ _ _ _ _ _ _ _ _ _ _]
      timeout: w17 -> [_ _ _ _ _ _ _ _ _ _ _ _ _ _ _ _ _ _]
      tunnel: w22 -> [_ w34 w36 w61 w72 _ _ _ _ _ _ _ _ _ _ _ _ _]
      tunnel: [_ w34 w36 w61 _ _ _ _ _ _ _ _ _ _ _ _ _ _] -> w15
      tunnel: [-1 w32 w41 w60 w69 w77 w81 w86 w90 w95 w99 w103 w107 w116 w118 w134 w136 w149] -> w21
      tunnel: w20 -> [_ _ _ _ _ _ _ _ _ _ _ _ _ _ _ _ _ _]
      tunnel: w19 -> [_ _ _ _ w64 _ _ _ _ _ _ _ _ _ _ _ _ _]
      tunnel: w18 -> [_ _ _ _ w63 _ _ _ _ _ _ _ _ _ _ _ _ _]
      tunnel: w17 -> [_ w32 w41 w60 w69 w77 w81 w86 w90 w95 w99 w103 w107 w116 w118 w134 w136 w149]
      tunnel: [string[] ["restore defaults", "clear"] string[] ["exit"] w37 string[] ["exit"] _ _ string[] ["ear"] _ _ string[] ["cal mic sens"] _ _ _ string[] ["cal mic sens"] _ string[] ["clear"] _ _] -> w16
      tunnel: [w24 w31 w38 w58 w66 w74 w79 w84 w88 w93 w97 w101 w105 w115 w117 w132 w135 w148] -> w13
      tunnel: w12 -> [w24 w31 w39 w58 w66 w74 w82 w85 w89 w94 w98 w102 w106 w114 w117 w132 w135 w148]
      event Timeout {
        w29 = TRUE ("Visible")
        n6 = event-data() -> ()  [unwired: 1 in, 1 out]
        n7 = global read "Calibration Globals.vi" "Probe Tube Folder"() -> (w28:path)
        n8 = call "SGDA-Initialize Hardware.vi"("Start PXI Server"=FALSE) -> ()  [unwired: 13 in, 2 out]
        n9 = call "isDir.vi"("path"=w28) -> ("is Dir?"=w27:bool)
        n10 = case shown="False" w27 {
          tunnel: w28 -> [w30 _]
          frame False {
            n11 = Create Folder(path (use dialog)=w30) -> ()  [unwired: 2 in, 3 out]
          }
          frame True {
          }
        }
        n12 = property on="RETURN" class="Bool"("Visible"=w29) -> ()  [unwired: 2 in, 2 out]
        n13 = property on="START" class="Bool"("Visible"=w29) -> ()  [unwired: 2 in, 2 out]
      }
      event Panel Close? {
        n14 = event-data() -> ()  [unwired: 1 in, 1 out]
        n15 = event-data("Discard?"=TRUE) -> ()  [unwired: 1 in, 1 out]
      }
      event Menu Selection (User) {
        n16 = event-data() -> ("ItemTag"=w40:string)  [unwired: 1 in]
        n17 = case shown="\"mmFileSave\"" w40 {
          tunnel: w39 -> [w42 w44 w46 w55 w57]
          tunnel: [w42 w44 w46 w55 w57] -> w38
          tunnel: [_ string[] ["restore params"] _ _ string[] ["exit"]] -> w37
          frame "", Default {
          }
          frame "mmFileRestore" {
          }
          frame "mmFileSave" {
            n18 = call "Config File Path.vi"("AppName"="CFTS") -> ("Default config file name"=w47:path)
            n19 = call "Write Anything.vi"("Section Name (Name of \"Anything\")"="PTCal" ("Section Name (Name of \"Type of Anything\")"), "Anything"=w46, "Path (dialog)"=w47) -> ("Error Out"=w45:errorcluster)  [unwired: 7 in, 1 out]
            n20 = case shown="Error" w45 {
              selector: w45 -> [_ w51]
              frame No Error {
                n21 = One Button Dialog(message="Defaults saved.") -> ()  [unwired: 1 in, 1 out]
              }
              frame Error {
                n22 = call "Error Handler.vi"("error in (no error)"=w51) -> ()  [unwired: 13 in, 2 out]
              }
            }
          }
          frame "mmFilePrint" {
            w54 = T17 1 items=["Complete front panel", "Visible portion of front panel", "Icon, description, panel and diagram", "Documentation: Using the panel", "Documentation: Using as a subVI", "Documentation: Complete", "Documentation: Custom"] ("contents (complete front panel)")
            n23 = control-ref of="This VI"() -> (w52:refnum<vi>)
            n24 = call-poly <vilib>:"Easy Print VI Panel or Documentation.vi"("layout options"="layout options", "contents (complete front panel)"=w54, "VI reference"=w52) -> ()  [unwired: 7 in, 2 out]
          }
          frame "mmFileExit" {
          }
        }
      }
      event "RETURN": Value Change {
        n25 = event-data() -> ()  [unwired: 1 in, 1 out]
      }
      event "START": Value Change {
        w71 = FALSE
        n26 = event-data() -> ()  [unwired: 1 in, 1 out]
        n27 = Unbundle By Name(w66) -> ("Ear"=w68:T13)
        n28 = call "CAL-Probe Tube Cal Path (L-R).vi"("Ear"=w68, "Right"=w64, "Left"=w63) -> ("Probe Tube Cal Path"=w67:path)  [unwired: 11 in, 1 out]
        n29 = Bundle("Probe Tube Cal Path"=w67, "Params"=w66) -> (w65:T18)  [unwired: 1 in]
        n30 = local write "Data tabs"(enum32{"Raw", "Calibration"}."Raw" ("Data tabs")) -> ()
        n31 = Send Notification(notification=w65, notifier=w72) -> ()  [unwired: 1 in, 2 out]
        n32 = property on="RETURN" class="Bool"("Visible"=w71) -> ()  [unwired: 2 in, 2 out]
        n33 = property on="START" class="Bool"("Visible"=w71) -> ()  [unwired: 2 in, 2 out]
        n34 = property on="Measure" class="Bool"("Visible"=w71) -> ()  [unwired: 2 in, 2 out]
        n35 = local write "Path"(path "" ("Path")) -> ()
      }
      event "finished": Value Change {
        w75 = TRUE
        n36 = event-data() -> ("NewVal"=w76:errorcluster)  [unwired: 1 in]
        n37 = call "Error Handler.vi"("error in (no error)"=w76) -> ()  [unwired: 13 in, 2 out]
        n38 = property on="START" class="Bool"("Visible"=w75) -> ()  [unwired: 2 in, 2 out]
        n39 = property on="RETURN" class="Bool"("Visible"=w75) -> ()  [unwired: 2 in, 2 out]
        n40 = property on="Measure" class="Bool"("Visible"=w75) -> ()  [unwired: 2 in, 2 out]
        n41 = call "Beeper.vi"() -> ()  [unwired: 5 in, 1 out]
        n42 = local write "Data tabs"(enum32{"Raw", "Calibration"}."Calibration" ("Data tabs")) -> ()
      }
      event Value Change {
        n43 = event-data() -> ()  [unwired: 1 in, 1 out]
        n44 = Bundle By Name(cluster=w82, "Ear"="Ear") -> (w79:T15)
      }
      event "Stimulus": Value Change {
        n45 = event-data() -> ()  [unwired: 1 in, 1 out]
        n46 = Bundle By Name(cluster=w85, "Stimulus"="Stimulus") -> (w84:T15)
      }
      event "Averages": Value Change {
        n47 = event-data() -> ()  [unwired: 1 in, 1 out]
        n48 = Bundle By Name(cluster=w89, "Averages"="Averages") -> (w88:T15)
      }
      event "Cal Mic Sens": Value Change {
        n49 = event-data() -> ("NewVal"=w91:dbl)  [unwired: 1 in]
        n50 = Bundle By Name(cluster=w94, "Cal Mic Sens"=w91) -> (w93:T15)
      }
      event "Cal Mic Gain (dB)": Value Change {
        n51 = event-data() -> ("NewVal"=w96:dbl)  [unwired: 1 in]
        n52 = Bundle By Name(cluster=w98, "Cal Mic Gain"=w96) -> (w97:T15)
      }
      event "Probe Mic Gain (dB)": Value Change {
        n53 = event-data() -> ("NewVal"=w100:dbl)  [unwired: 1 in]
        n54 = Bundle By Name(cluster=w102, "Probe Mic Gain"=w100) -> (w101:T15)
      }
      event "Correction curve": Value Change {
        n55 = event-data() -> ()  [unwired: 1 in, 1 out]
        n56 = Bundle By Name(cluster=w106, "Correction"="Correction curve") -> (w105:T15)
      }
      event "Measure": Value Change {
        n57 = event-data() -> ()  [unwired: 1 in, 1 out]
        n58 = Unbundle By Name(w114) -> ("Cal Mic Sens"=w111:dbl)
        n59 = call "Cxns-Get Connections File Path.vi"() -> ("Path Out"=w110:path)  [unwired: 1 in]
        n60 = call "Equip-Get Device (TDT).vi"("Path In"=w110) -> ("TDT-Device Config"=w109:T19)  [unwired: 12 in, 2 out]
        n61 = call "Cal Mic Sensitivity (TDT).vi"("Device Config"=w109, "User ID"="User ID", "Mic Sens (dB V/SPL) in"=w111) -> ("Mic Sens (dB V/SPL)"=w108:dbl)  [unwired: 8 in]
        n62 = Bundle By Name(cluster=w114, "Cal Mic Sens"=w108) -> (w115:T15)
        n63 = local write "Cal Mic Sens"(w108) -> ()
      }
      event "Open Button": Value Change {
        n64 = event-data() -> ()  [unwired: 1 in, 1 out]
        n65 = global read "Calibration Globals.vi" "Probe Tube Folder"() -> (w119:path)
        n66 = control-ref of="PT phase"() -> (w123:refnum<vi>)
        n67 = control-ref of="PT mag"() -> (w124:refnum<vi>)
        n68 = call "File Dialog"("start path"=w119, "pattern (all files)"="*.calib", "pattern label"="Calibration files") -> ("selected path"=w125:path, "cancelled"=w126:bool, "error out"=w122:errorcluster)  [unwired: 9 in, 1 out]
        n69 = case shown="False" w126 {
          tunnel: w125 -> [w127 _]
          tunnel: w124 -> [w129 _]
          tunnel: w123 -> [w128 _]
          tunnel: w122 -> [w131 _]
          frame False {
            n70 = call "CAL-Plot data.vi"("Path"=w127, "Mag graph"=w129, "Phase graph"=w128, "error in (no error)"=w131) -> ("error out"=w130:errorcluster)  [unwired: 10 in, 1 out]
            n71 = local write "Path"(w127) -> ()
            n72 = call "Error Handler.vi"("error in (no error)"=w130) -> ()  [unwired: 13 in, 2 out]
          }
          frame True {
          }
        }
      }
      event "Clear Button": Value Change {
        n73 = event-data() -> ()  [unwired: 1 in, 1 out]
      }
      event "Smooth Button": Value Change {
        n74 = event-data() -> ()  [unwired: 1 in, 1 out]
        n75 = local read "Path"() -> (w139:path)
        n76 = control-ref of="PT mag"() -> (w138:refnum<vi>)
        n77 = control-ref of="PT phase"() -> (w137:refnum<vi>)
        n78 = call "Calibration Smoothing Tool.vi"("Path In"=w139) -> ("Smoothed?"=w140:bool)  [unwired: 10 in]
        n79 = case shown="True" w140 {
          tunnel: w139 -> [_ w143]
          tunnel: w138 -> [_ w145]
          tunnel: w137 -> [_ w144]
          frame False {
          }
          frame True {
            w147 = cluster{"PTC Mag":dbl[], "PTC Phase":dbl[]}[] [] ("PT mag graph")
            n80 = property on="Property Node" class="XYGraph (strict)"(reference=w144, "Value"=w147) -> (reference out=w141:refnum<vi>)  [unwired: 1 in, 1 out]
            n81 = property on="Property Node" class="XYGraph (strict)"(reference=w145, "Value"=w147, "Legend Visible"=FALSE ("Legend:Visible")) -> (reference out=w142:refnum<vi>)  [unwired: 1 in, 1 out]
            n82 = call "CAL-Plot data.vi"("Path"=w143, "Mag graph"=w142, "Phase graph"=w141) -> ()  [unwired: 11 in, 2 out]
          }
        }
      }
      event "Validate Button": Value Change {
        n83 = event-data() -> ()  [unwired: 1 in, 1 out]
        n84 = local read "Probe Mic Gain (dB)"() -> (w153:dbl)
        n85 = local read "Cal Mic Sens"() -> (w151:dbl)
        n86 = local read "Cal Mic Gain (dB)"() -> (w152:dbl)
        n87 = local read "Path"() -> (w156:path)
        n88 = local read "Ear"() -> (w150:T13)
        n89 = call "FileIO-File or Folder Exists.vi"("path"=w156) -> ("Exists?"=w155:bool, "dup path"=w154:path)  [unwired: 7 in, 2 out]
        n90 = case shown="True" w155 {
          tunnel: w154 -> [_ w161]
          tunnel: w153 -> [_ w160]
          tunnel: w152 -> [_ w159]
          tunnel: w151 -> [_ w158]
          tunnel: w150 -> [_ w157]
          frame False {
          }
          frame True {
            n91 = call "Cal Validation.vi"("Path In"=w161, "Probe Mic Gain (dB)"=w160, "Cal Mic Gain (dB)"=w159, "Cal Mic Sens (dB)"=w158, "Ear"=w157) -> ()  [unwired: 11 in]
          }
        }
      }
    }
    n92 = while {
      shift-right: [w167] -> _
      shift-left: w16 -> [w170]
      tunnel: w15 -> [w165]
      tunnel: [w164] -> w14
      shift-right: [w162] -> w11
      shift-left: w13 -> [w163]
      stop <- w166 stop-if-true
      n93 = Delete From Array(array=w170) -> (deleted portion=w168:string, array with subset deleted=w169:string[])  [unwired: 2 in]
      n94 = case shown="\"cal mic sens\"" w168 {
        tunnel: w169 -> [w172 w177 w188 w206 w214 w222 w226]
        tunnel: [w172 w177 w182 w197 w214 w222 w226] -> w167
        tunnel: w165 -> [_ w176 _ _ _ _ _]
        tunnel: [_ TRUE _ _ _ _ _] -> w164
        tunnel: w163 -> [w171 w174 w184 w205 w213 w221 w223]
        tunnel: [w171 w174 w183 w205 w213 w221 w223] -> w162
        frame "", Default {
        }
        frame "exit" {
          n95 = Release Notifier(notifier=w176) -> ()  [unwired: 2 in, 3 out]
          n96 = call "SGDA-Close Hardware.vi"("Stop PXI Server (T)"=FALSE) -> ()  [unwired: 6 in, 1 out]
        }
        frame "restore defaults" {
          n97 = call "Config File Path.vi"("AppName"="CFTS") -> ("Default config file name"=w178:path)
          n98 = call "Read Anything.vi"("Type of Anything"=w184, "Section Name (Name of \"Type of Anything\")"="PTCal" ("Section Name (Name of \"Type of Anything\")"), "Path (dialog)"=w178) -> ("Error Out"=w186:errorcluster, "Found?"=w187:bool, "Anything"=w185:variant)  [unwired: 6 in]
          n99 = case shown="False" w187 {
            tunnel: w186 -> [_ w193]
            tunnel: w185 -> [_ w194]
            tunnel: w184 -> [w190 w192]
            tunnel: [w189 w191] -> w183
            frame False {
              n100 = call "ACal-Update Probe Tube Parameters.vi"("Params in"=w190) -> ("Params out"=w189:T15)  [unwired: 14 in]
            }
            frame True {
              n101 = Variant To Data(error in=w193, type=w192, Variant=w194) -> (data=w191:T15)  [unwired: 1 out]
            }
          }
          n102 = Build Array (concatenate)(w188, "show") -> (w182:string[])
        }
        frame "show" {
          n103 = Unbundle By Name(w205) -> ("Ear"=w204:T13, "Stimulus"=w203:T16, "Averages"=w202:i32, "Cal Mic Gain"=w201:dbl, "Probe Mic Gain"=w200:dbl, "Cal Mic Sens"=w199:dbl, "Correction"=w198:path)
          n104 = local write "Ear"(w204) -> ()
          n105 = local write "Stimulus"(w203) -> ()
          n106 = local write "Averages"(w202) -> ()
          n107 = local write "Cal Mic Gain (dB)"(w201) -> ()
          n108 = local write "Probe Mic Gain (dB)"(w200) -> ()
          n109 = local write "Cal Mic Sens"(w199) -> ()
          n110 = local write "Correction curve"(w198) -> ()
          n111 = Build Array (concatenate)(w206, "ear", "cal mic sens") -> (w197:string[])
        }
        frame "ear" {
          n112 = Unbundle By Name(w213) -> ("Ear"=w209:T13)
          n113 = local read "Right"() -> (w208:string)
          n114 = local read "Left"() -> (w207:string)
          n115 = Equal?(x=Left-Right_ring."Right", y=w209) -> (x = y?=w211:bool)
          n116 = Select(t=w208, s=w211, f=w207) -> (s? t:f=→"Acoustic System ID":string)
        }
        frame "cal mic sens" {
          n117 = Unbundle By Name(w221) -> ("Cal Mic Sens"=w215:dbl)
          n118 = call-poly "dB to Linear.vi"("dB"=w215) -> ("linear"=w216:dbl)
          n119 = Divide(x=w216, y=2e-05) -> (x/y=w218:dbl)
          n120 = Multiply(x=w218, y=1000.0) -> (x*y=→"(mV/Pa)":dbl)
        }
        frame "clear" {
          w225 = cluster{"PTC Mag":dbl[], "PTC Phase":dbl[]}[] [] ("PT mag graph")
          n121 = property on="PT mag" class="XYGraph (strict)"("Value"=w225, "Legend Visible"=FALSE ("Legend:Visible")) -> ()  [unwired: 2 in, 2 out]
          n122 = property on="PT phase" class="XYGraph (strict)"("Value"=w225) -> ()  [unwired: 2 in, 2 out]
        }
      }
      n123 = Empty Array?(array=w167) -> (empty?=w166:bool)
    }
  }
  n124 = while {
    tunnel: w10 -> [w231]
    stop <- w230 stop-if-true
    # "MEASUREMENT THREAD"
    n125 = Wait on Notification(notifier=w231, ignore previous (F)=TRUE) -> (notification=w229:cluster{path, "Params":T15}, error out=w230:errorcluster)  [unwired: 2 in, 2 out]
    n126 = Unbundle(w229) -> (w228:path, "Params"=w227:T15)
    n127 = case shown="No Error" w230 {
      tunnel: w228 -> [w241 _]
      tunnel: w227 -> [w238 _]
      frame No Error {
        # "cal mic index"
        # "frequency spacing"
        # "sampling interval"
        # "running sum"
        n128 = control-ref of="Mic mag"() -> (w259:refnum<vi>)
        n129 = Unbundle By Name(w238) -> ("Stimulus"=w242:T16)
        n130 = Unbundle By Name(w238) -> ("Ear"=w240:T13)
        n131 = Unbundle By Name(w238) -> ("Averages"=w239:i32)
        n132 = call "CPT-Config.vi"("Cal Stimulus"=w242, "Ear"=w240, "Mic mag graph ref"=w259) -> ("Stimulus waveform"=→"Stimulus graph":cluster{i32, dbl, dbl[]}, "Mic Avg"=w268:dbl[][], "dt (ms)"=w266:dbl, "df (Hz)"=w267:dbl, "Cal mic index"=w261:i16, "error out"=w269:errorcluster)  [unwired: 5 in, 2 out]
        n133 = call "SGDA-Start.vi"("error in (no error)"=w269) -> ("error out"=w258:errorcluster)  [unwired: 6 in]
        n134 = while {
          tunnel: w258 -> [w291]
          tunnel: [w271] -> w257
          tunnel: w239 -> [w289]
          shift-right: [w287] -> _
          shift-left: w268 -> [w288]
          tunnel: [w286] -> _
          tunnel: 5 -> [w285]
          tunnel: w267 -> [w280]
          tunnel: [w279] -> w264
          tunnel: [w278] -> w263
          tunnel: w266 -> [w277]
          tunnel: [w276] -> w262
          i -> [w290]
          stop <- w281 stop-if-true
          # "Perform these operations every Nth\naverage, or when we're about to stop\n(i.e. on the last average)."
          # "running avg"
          # "running sum"
          n135 = call "SGDA-Read Data.vi"("error in (no error)"=w291) -> ("AI Waveforms"=w274:dbl[][], "error out"=w271:errorcluster)  [unwired: 13 in]
          n136 = Increment(x=w290) -> (x+1=w275:i32)
          "Acquired" <- w275
          n137 = Equal?(x=w275, y=w289) -> (x = y?=w272:bool)
          n138 = Quotient & Remainder(x=w275, y=w285) -> (x-y*floor(x/y)=w284:i32)  [unwired: 1 out]
          n139 = Add(x=w274, y=w288) -> (x+y=w287:dbl[][])
          n140 = Equal To 0?(x=w284) -> (x = 0?=w282:bool)
          n141 = Compound Arithmetic op=OR(w271, w272, "STOP") -> (w281:bool)
          n142 = Or(x=w282, y=w281) -> (x .or. y?=w283:bool)
          n143 = Divide(x=w287, y=w275) -> (x/y=w286:dbl[][])
          n144 = case shown="True" w283 {
            tunnel: w286 -> [_ w295]
            tunnel: w280 -> [_ w292]
            tunnel: [_ w297] -> w279
            tunnel: [_ w296] -> w278
            tunnel: w277 -> [_ w294]
            tunnel: [_ w292] -> w276
            frame False {
            }
            frame True {
              # "phase"
              # "magnitude"
              n145 = call-poly "Create Waveform Cluster.vi"("dx"=w294, "Array"=w295) -> ("waveform cluster"=→"Mic signals":cluster{"offset":dbl, "dx":dbl, "Y":dbl[][]})  [unwired: 3 in]
              n146 = call-poly "FFT x(t) to dB,Degrees.vi"("X(t)"=w295) -> ("+Freq Phase of FFT (degrees)"=w296:dbl[][], "+Freq. Mag of FFT (dB rms)"=w297:dbl[][])  [unwired: 9 in]
              n147 = call-poly "Create Waveform Cluster.vi"("dx"=w292, "Array"=w297) -> ("waveform cluster"=→"Mic mag":cluster{"offset":dbl, "dx":dbl, "Y":dbl[][]})  [unwired: 3 in]
              n148 = call-poly "Create Waveform Cluster.vi"("dx"=w292, "Array"=w296) -> ("waveform cluster"=→"Mic phase":cluster{"offset":dbl, "dx":dbl, "Y":dbl[][]})  [unwired: 3 in]
            }
          }
          n149 = Wait (ms)(milliseconds to wait=u32 5) -> ()  [unwired: 1 out]
        }
        n150 = call "SGDA-Stop.vi"("Clear ActiveX (F)"=TRUE, "error in (no error)"=w257) -> ("error out"=w265:errorcluster)  [unwired: 13 in]
        n151 = Unbundle By Name(w238) -> ("Cal Mic Sens"=w237:dbl, "Cal Mic Gain"=w236:dbl, "Probe Mic Gain"=w235:dbl, "Correction"=w234:path)
        n152 = call "CPT-Compute PTC.vi"("Mag"=w264, "Phase"=w263, "df (Hz)"=w262, "Cal mic index"=w261, "error in (no error)"=w265, "Cal Mic Sensitivity \n(dB V/SPL)"=w237, "Cal Mic Gain (dB)"=w236, "Probe Mic Gain (dB)"=w235) -> ("PTC Mag"=w250:dbl[], "PTC Phase"=w248:dbl[], "Frequency"=w246:dbl[], "error out"=w245:errorcluster)  [unwired: 4 in]
        n153 = control-ref of="PT mag"() -> (w254:refnum<vi>)
        n154 = control-ref of="PT phase"() -> (w253:refnum<vi>)
        n155 = call "Cal-Apply Microphone Correction.vi"("PTC Mag in"=w250, "PTC Phase in"=w248, "Frequency in"=w246, "Correction curve"=w234, "error in (no error)"=w245) -> ("PTC Mag out"=w251:dbl[], "PTC Phase out"=w249:dbl[], "Frequency out"=w247:dbl[], "error out"=w244:errorcluster)  [unwired: 7 in]
        n156 = call "CAL-Save data.vi"("Mag"=w251, "Phase"=w249, "Frequency"=w247, "path"=w241, "error in (no error)"=w244, "Cal Stimulus"=w242) -> ("new file path"=w252:path, "error out"=w255:errorcluster)  [unwired: 8 in]
        "Path" <- w252
        n157 = call "CAL-Plot data.vi"("Path"=w252, "Mag graph"=w254, "Phase graph"=w253, "error in (no error)"=w255) -> ("error out"=w243:errorcluster)  [unwired: 10 in, 1 out]
        n158 = property on="finished" class="Clust (strict)"("Val(Sgnl)"=w243) -> ()  [unwired: 2 in, 2 out]
      }
      frame Error {
      }
    }
  }
